vi "Set Tree Symbols.vi"(8 "error in (no error)":errorcluster, 11 "Process Builder View in":refnum<class "Process Builder View.lvclass">) -> (0 "error out":errorcluster, 3 "Process Builder View out":refnum<class "Process Builder View.lvclass">)   [LabVIEW 2019, in "Process Builder View.lvclass"]
uses:
  <vilib>/gpm_packages/@cs/Car-wash/Source/Process Builder View/Process Builder View.lvclass
  C:/Program Files/National Instruments/LabVIEW 2019/vi.lib/gpm_packages/@cs/Test-executive-builder/Source/Test Executive Builder View/Test Executive Builder View/Test Executive Builder View.lvclass
  <vilib>/gpm_packages/@cs/Test-executive-builder/Source/Test Executive Builder View/Test Executive Builder View/Test Executive Builder View.lvclass/Test Executive Builder View.ctl
  <vilib>/gpm_packages/@cs/Test-executive-builder/Source/Test Executive Builder View/Test Executive Builder View/Test Executive Builder View.lvclass
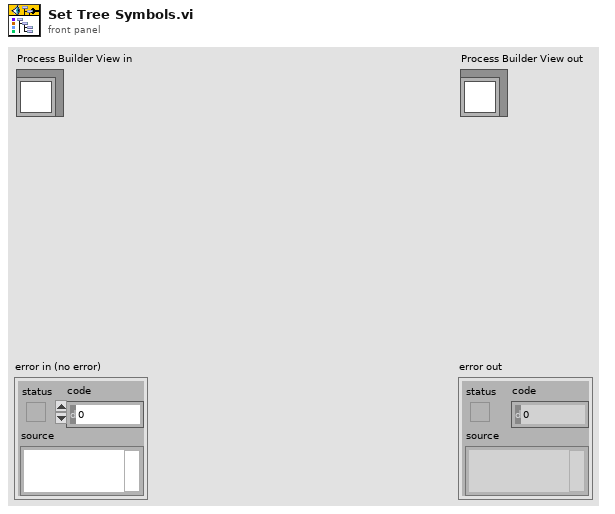
[diagram p1: front panel]
types:
  T1 = typedef "imagedata.ctl" = cluster{"image type":i32, "image depth":i32, "image":u8[], "mask":u8[], "colors":u32[], "Rectangle":cluster{"left":i16, "top":i16, "right":i16, "bottom":i16}}
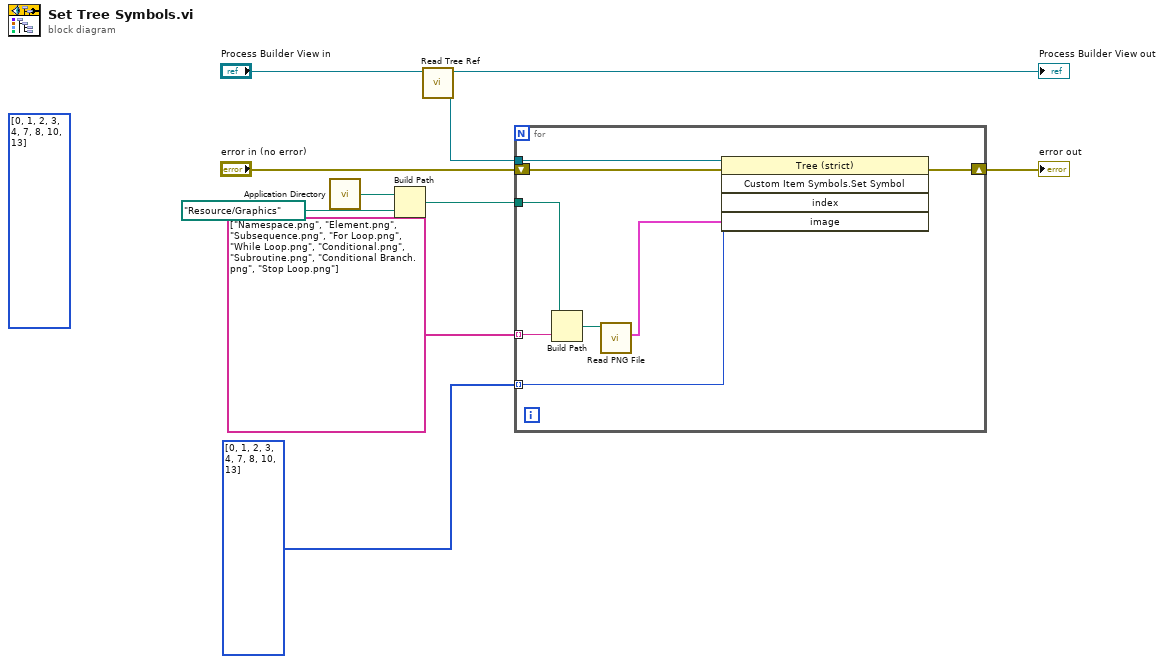
[diagram p0: block diagram]
diagram:
  (unwired) i32[] [0, 1, 2, 3, 4, 7, 8, 10, 13]
  n1 = call <vilib>:"Application Directory.vi"() -> ("Application Directory"=w5:path)
  n2 = Build Path(base path=w5, name or relative path=path "Resource/Graphics") -> (appended path=w1:path)
  n3 = call <vilib>:"Read Tree Ref.vi"("Test Executive Builder View in"="Process Builder View in") -> ("Tree Ref"=w10:refnum<vi>, "Test Executive Builder View out"=→"Process Builder View out":refnum<class "Process Builder View.lvclass">)  [unwired: 9 in]
  n4 = for {
    tunnel: w10 -> [w18]
    shift-right: [w16] -> w6
    shift-left: "error in (no error)" -> [w17]
    tunnel: i32[] [0, 1, 2, 3, 4, 7, 8, 10, 13] -> [w11] mode=indexing
    tunnel: string[] ["Namespace.png", "Element.png", "Subsequence.png", "For Loop.png", "While Loop.png", "Conditional.png", "Subroutine.png", "Conditional Branch.png", "Stop Loop.png"] -> [w13] mode=indexing
    tunnel: w1 -> [w14]
    n5 = Build Path(base path=w14, name or relative path=w13) -> (appended path=w15:path)
    n6 = call <vilib>:"Read PNG File.vi"("path to PNG file"=w15) -> ("image data"=w12:T1)  [unwired: 8 in, 2 out]
    n7 = invoke class="Tree (strict)" method="Custom Item Symbols.Set Symbol"(reference=w18, error in=w17, "index"=w11, "image"=w12) -> (error out=w16:errorcluster)  [unwired: 1 in, 4 out]
  }
  "error out" <- w6
